vi "PE Get Status Str.vi"(8 "error in (no error)":errorcluster, 11 "code":i32) -> (0 "error out":errorcluster, 3 "function return":string)   [LabVIEW 2017, in "PE_Filter_SDK.lvlib"]
doc: "PEFILTERSDK_API const char* PE_GetStatusStr(PE_STATUS code);"
uses:
  PE_Filter_SDK.lvlib
  PE_Filter_SDK.dll
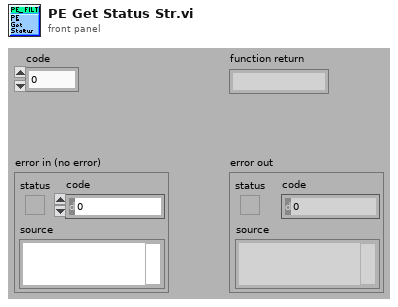
[diagram p1: front panel]
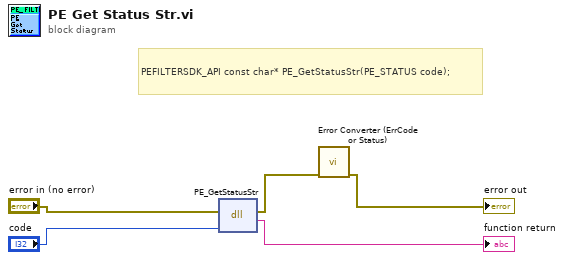
[diagram p0: block diagram]
diagram:
  # "PEFILTERSDK_API const char* PE_GetStatusStr(PE_STATUS code);"
  n1 = dll-call lib="D:/working_directory/SDK LLTF/trunk_commit/examples/PE_Filter_SDK/PE_Filter_SDK.*" fn="PE_GetStatusStr"(error in="error in (no error)", "code"="code") -> (error out=w2:errorcluster, →"function return":string)  [unwired: 3 in, 1 out]
  n2 = call "Error Converter (ErrCode or Status).vi"("error in (no error)"=w2) -> ("error out"=→"error out":errorcluster)  [unwired: 10 in]
